vi "调试画面.vi"() -> ()   [LabVIEW 2016, in "main.lvlib"]
uses:
  main.lvlib
  elevator/elevator.lvlib
  DAM395CF/DAM395CF.lvlib
  EXO2/EXO2.lvlib
  bbe/bbe.lvlib
panel:
  in  "设置初值":bool
  in  "保存数据":bool
  in  "EXO2停止":bool
  in  "EXO2启动":bool
  in  "定位位置":dbl format="%#_6f m"
  out "仪器位置":dbl format="%#_6f m"
  in  "仪器通电":bool
  in  "定位":bool
  in  "停止按钮":bool
  in  "向下按钮":bool
  in  "向上按钮":bool
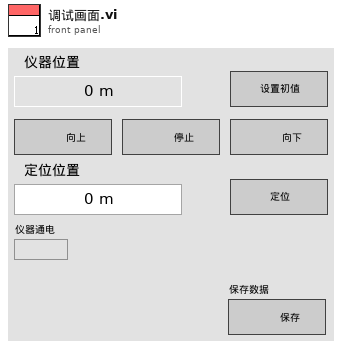
[diagram p1: front panel]
types:
  T1 = typedef "剖面数据_EXO2.ctl" = cluster{"时间":timestamp, "测量模式":string, "数据类型":string, "数据标识":string, "湖面水深":sgl, "缆绳下放长度":sgl, "层数":u16, "row":u16, "水温":sgl, "比电导率":sgl, "电导率":sgl, "盐度":sgl, "总溶解固体":sgl, "pH":sgl, "pHmV":sgl, "ORP":sgl, "饱和度":sgl, "DO":sgl, "浊度":sgl, "叶绿素a":sgl, "水深":sgl}
  T2 = typedef "剖面数据_bbe_NAQDO.ctl" = cluster{"时间":timestamp, "测量模式":string, "数据类型":string, "数据标识":string, "湖面水深":sgl, "缆绳下放长度":sgl, "层数":u16, "row":u16, "水温":sgl, "DO":sgl, "饱和度":sgl, "绿藻":sgl, "蓝藻":sgl, "硅甲藻":sgl, "隐藻":sgl, "透光率":sgl, "水深":sgl}
  T3 = enum16{"open", "poll", "close", "run", "stop", "shutdown"}
  T4 = cluster{"Time":timestamp, "Temp":dbl, "SpCond":dbl, "Cond":dbl, "Sal":dbl, "TDS":dbl, "pH":dbl, "pH mV":dbl, "orp":dbl, "ODO %":dbl, "ODO mg/L":dbl, "Turb":dbl, "Chl":dbl, "Depth":dbl}
  T5 = cluster{"时间":timestamp, "Temp [℃]":dbl, "Green Algae [μg/L]":dbl, "Bluegreen [μg/L]":dbl, "Diatoms [μg/L]":dbl, "Cryptophyta [μg/L]":dbl, "Transmission [%]":dbl, "Depth [m]":dbl}
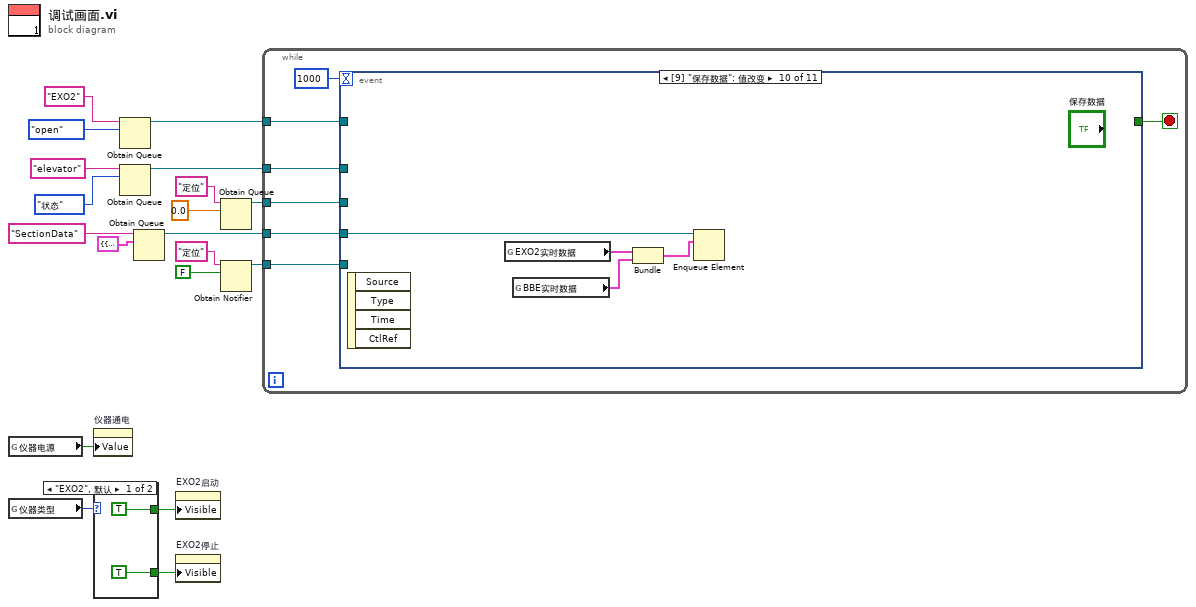
[diagram p0: block diagram]
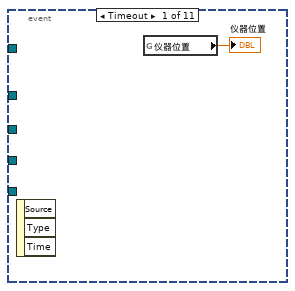
[diagram p3: hidden frame]
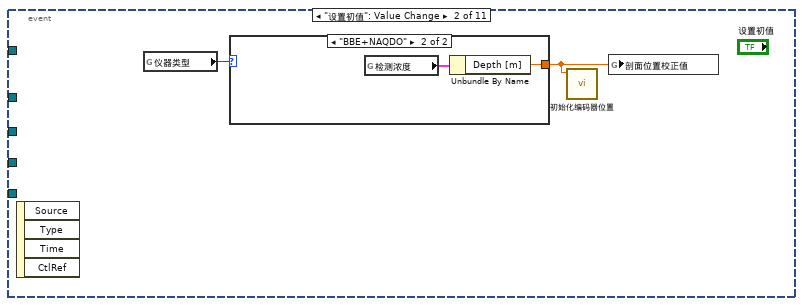
[diagram p4: hidden frame]
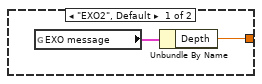
[diagram p5: hidden frame]
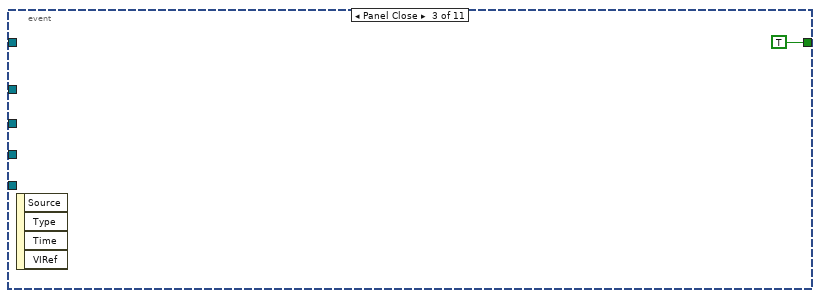
[diagram p6: hidden frame]
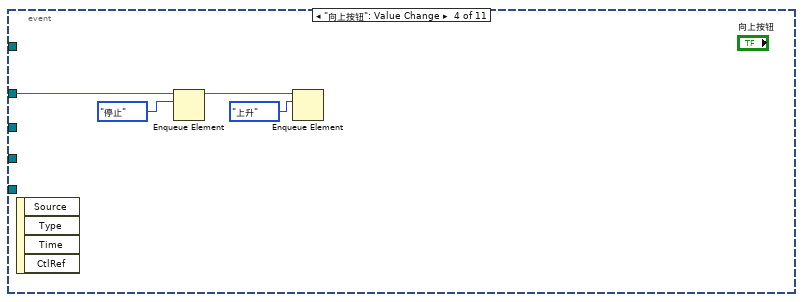
[diagram p7: hidden frame]
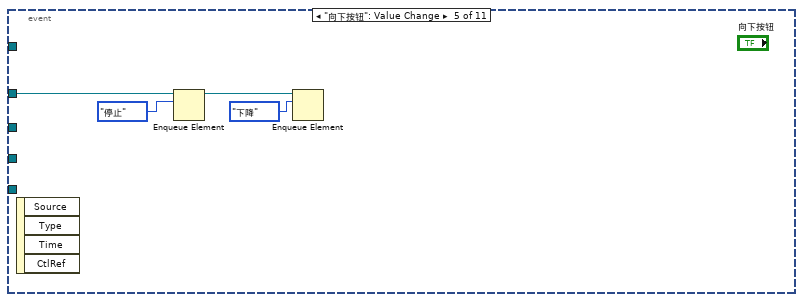
[diagram p8: hidden frame]
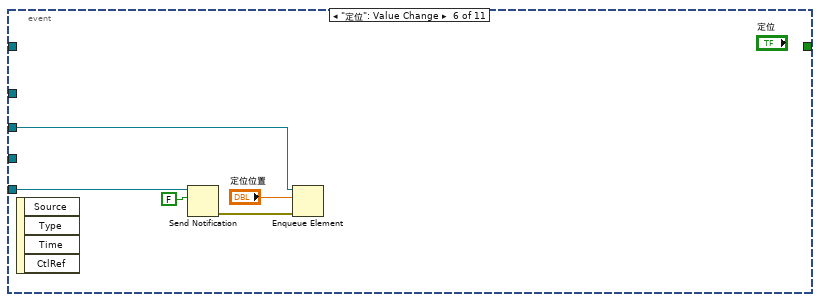
[diagram p9: hidden frame]
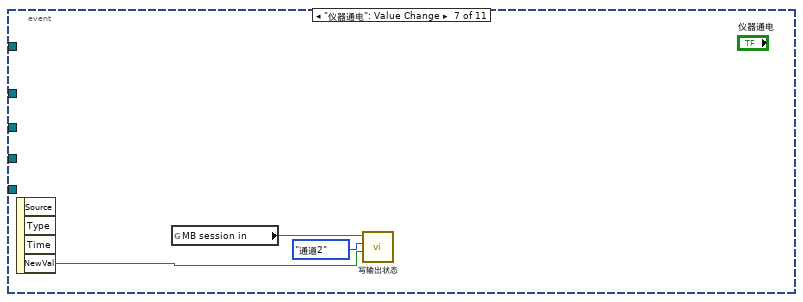
[diagram p10: hidden frame]
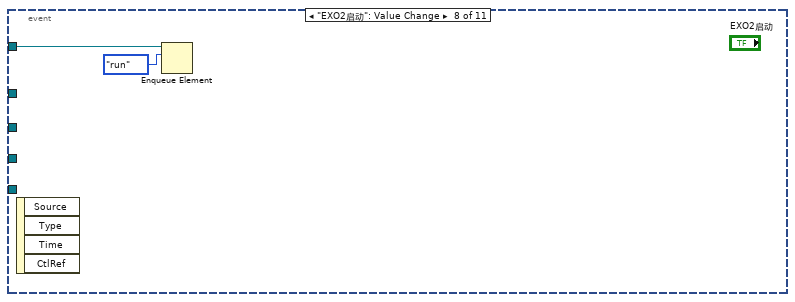
[diagram p11: hidden frame]
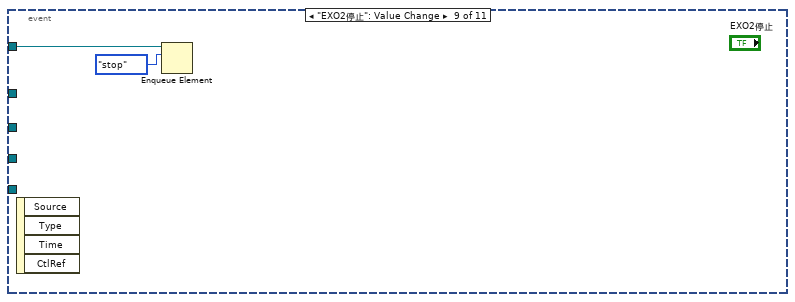
[diagram p12: hidden frame]
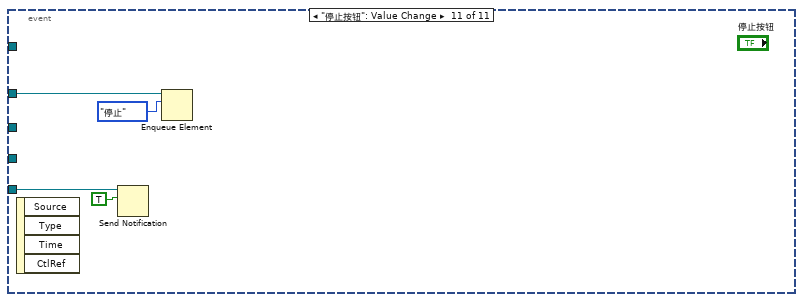
[diagram p13: hidden frame]
diagram:
  n1 = global read "全局非断电保持变量.vi" "仪器电源"() -> (w7:bool)
  n2 = global read "全局断电保存变量.vi" "仪器类型"() -> (w6:enum16{"EXO2", "BBE+NAQDO"})
  n3 = property on="仪器通电" class="Bool (严格)"("Value"=w7) -> ()  [unwired: 2 in, 2 out]
  n4 = case shown="\"EXO2\", 默认" w6 {
    tunnel: [TRUE _] -> w5
    tunnel: [TRUE _] -> w4
    frame "EXO2", Default {
    }
    frame "BBE+NAQDO" {
    }
  }
  n5 = Obtain Queue(name (unnamed)="EXO2" ("名称（未命名）"), element data type=T3."open" ("枚举")) -> (queue out=w14:refnum<queue>)  [unwired: 3 in, 2 out]
  n6 = Obtain Queue(name (unnamed)="elevator" ("名称（未命名）"), element data type=enum16{"状态", "上升", "下降", "停止"}."状态" ("枚举")) -> (queue out=w17:refnum<queue>)  [unwired: 3 in, 2 out]
  n7 = Obtain Queue(name (unnamed)="SectionData" ("名称（未命名）"), element data type=cluster{"EXO2 message":T1, "bbe message":T2} {"EXO2 message"={"时间"=timestamp(0 s since 1904-01-01), "测量模式"="水样测试", "数据类型"="N", "数据标识"="N", "湖面水深"=0.0, "缆绳下放长度"=0.0, "层数"=0, "row"=0, "水温"=0.0, "比电导率"=0.0, "电导率"=0.0, "盐度"=0.0, "总溶解固体"=0.0, "pH"=0.0, "pHmV"=0.0, "ORP"=0.0, "饱和度"=0.0, "DO"=0.0, "浊度"=0.0, "叶绿素a"=0.0, "水深"=0.0}, "bbe message"={"时间"=timestamp(0 s since 1904-01-01), "测量模式"="水样测试", "数据类型"="N", "数据标识"="N", "湖面水深"=0.0, "缆绳下放长度"=0.0, "层数"=0, "row"=0, "水温"=0.0, "DO"=0.0, "饱和度"=0.0, "绿藻"=0.0, "蓝藻"=0.0, "硅甲藻"=0.0, "隐藻"=0.0, "透光率"=0.0, "水深"=0.0}} ("簇")) -> (queue out=w1:refnum<queue>)  [unwired: 3 in, 2 out]
  n8 = property on="EXO2启动" class="Bool"("Visible"=w5) -> ()  [unwired: 2 in, 2 out]
  n9 = property on="EXO2停止" class="Bool"("Visible"=w4) -> ()  [unwired: 2 in, 2 out]
  n10 = Obtain Queue(name (unnamed)="定位" ("名称（未命名）"), element data type=0.0) -> (queue out=w8:refnum<queue>)  [unwired: 3 in, 2 out]
  n11 = Obtain Notifier(name (unnamed)="定位" ("名称（未命名）"), notification data type=FALSE) -> (notifier out=w9:refnum<notifier>)  [unwired: 2 in, 2 out]
  n12 = while {
    tunnel: w17 -> [w27]
    tunnel: w14 -> [w25]
    tunnel: w9 -> [w24]
    tunnel: w8 -> [w23]
    tunnel: w1 -> [w22]
    stop <- w28 stop-if-true
    n13 = event shown="[9] \"保存数据\": 值改变" {
      selector: _ -> [_ _ _ _ _ _ _ _ _ _ _]
      dyn-events: _ -> [_ _ _ _ _ _ _ _ _ _ _]
      timeout: 1000 -> [_ _ _ _ _ _ _ _ _ _ _]
      tunnel: [_ _ TRUE _ _ _ _ _ _ _ _] -> w28
      tunnel: w27 -> [_ _ _ w40 w44 _ _ _ _ _ w64]
      tunnel: w25 -> [_ _ _ _ _ _ _ w54 w56 _ _]
      tunnel: w24 -> [_ _ _ _ _ w47 _ _ _ _ w62]
      tunnel: w23 -> [_ _ _ _ _ w49 _ _ _ _ _]
      tunnel: w22 -> [_ _ _ _ _ _ _ _ _ w60 _]
      event Timeout {
        n14 = event-data() -> ()  [unwired: 1 in, 3 out]
        n15 = global read "全局非断电保持变量.vi" "仪器位置"() -> (→"仪器位置":dbl)
      }
      event "设置初值": Value Change {
        n16 = event-data() -> ()  [unwired: 1 in, 4 out]
        n17 = global read "全局断电保存变量.vi" "仪器类型"() -> (w30:enum16{"EXO2", "BBE+NAQDO"})
        n18 = case shown="\"BBE+NAQDO\"" w30 {
          tunnel: [w33 w34] -> w31
          frame "EXO2", Default {
            n19 = global read "EXO2全局变量.vi" "EXO message"() -> (w32:T4)
            n20 = Unbundle By Name(w32) -> ("Depth"=w33:dbl)
          }
          frame "BBE+NAQDO" {
            n21 = global read "过程变量.vi" "检测浓度"() -> (w35:T5)
            n22 = Unbundle By Name(w35) -> ("Depth [m]"=w34:dbl)
          }
        }
        n23 = call "初始化编码器位置.vi"("原始位置"=w31) -> ()  [unwired: 10 in, 1 out]
        n24 = global write "全局断电保存变量.vi" "剖面位置校正值"(w31) -> ()
      }
      event Panel Close {
        n25 = event-data() -> ()  [unwired: 1 in, 4 out]
      }
      event "向上按钮": Value Change {
        n26 = event-data() -> ()  [unwired: 1 in, 4 out]
        n27 = Enqueue Element(queue=w40, element=enum16{"状态", "上升", "下降", "停止"}."停止" ("元素")) -> (queue out=w37:refnum<queue>)  [unwired: 2 in, 2 out]
        n28 = Enqueue Element(queue=w37, element=enum16{"状态", "上升", "下降", "停止"}."上升" ("元素")) -> ()  [unwired: 2 in, 3 out]
      }
      event "向下按钮": Value Change {
        n29 = event-data() -> ()  [unwired: 1 in, 4 out]
        n30 = Enqueue Element(queue=w44, element=enum16{"状态", "上升", "下降", "停止"}."停止" ("元素")) -> (queue out=w41:refnum<queue>)  [unwired: 2 in, 2 out]
        n31 = Enqueue Element(queue=w41, element=enum16{"状态", "上升", "下降", "停止"}."下降" ("元素")) -> ()  [unwired: 2 in, 3 out]
      }
      event "定位": Value Change {
        n32 = event-data() -> ()  [unwired: 1 in, 4 out]
        n33 = Send Notification(notification=FALSE ("通知"), notifier=w47) -> (error out=w45:errorcluster)  [unwired: 1 in, 1 out]
        n34 = Enqueue Element(queue=w49, element="定位位置", error in (no error)=w45) -> ()  [unwired: 1 in, 3 out]
      }
      event "仪器通电": Value Change {
        n35 = event-data() -> ("NewVal"=w50:bool)  [unwired: 1 in, 3 out]
        n36 = global read "elevator 全局变量.vi" "MB session in"() -> (w51:refnum<class "MB_Master.lvclass">)
        n37 = call "写输出状态.vi"("value"=w50, "通道"=enum16{"通道0", "通道1", "通道2", "通道3"}."通道2", "MB session in"=w51) -> ()  [unwired: 7 in, 2 out]
      }
      event "EXO2启动": Value Change {
        n38 = event-data() -> ()  [unwired: 1 in, 4 out]
        n39 = Enqueue Element(queue=w54, element=T3."run" ("元素")) -> ()  [unwired: 2 in, 3 out]
      }
      event "EXO2停止": Value Change {
        n40 = event-data() -> ()  [unwired: 1 in, 4 out]
        n41 = Enqueue Element(queue=w56, element=T3."stop" ("元素")) -> ()  [unwired: 2 in, 3 out]
      }
      event "保存数据": Value Change {
        n42 = event-data() -> ()  [unwired: 1 in, 4 out]
        n43 = global read "全局非断电保持变量.vi" "EXO2实时数据"() -> (w59:T1)
        n44 = global read "全局非断电保持变量.vi" "BBE实时数据"() -> (w58:T2)
        n45 = Bundle("EXO2实时数据"=w59, "BBE实时数据"=w58) -> (w57:cluster{"EXO2实时数据":T1, "BBE实时数据":T2})  [unwired: 1 in]
        n46 = Enqueue Element(queue=w60, element=w57) -> ()  [unwired: 2 in, 3 out]
      }
      event "停止按钮": Value Change {
        n47 = event-data() -> ()  [unwired: 1 in, 4 out]
        n48 = Send Notification(notification=TRUE ("通知"), notifier=w62) -> ()  [unwired: 1 in, 2 out]
        n49 = Enqueue Element(queue=w64, element=enum16{"状态", "上升", "下降", "停止"}."停止" ("元素")) -> ()  [unwired: 2 in, 3 out]
      }
    }
  }
